vi "AC_Disconnect_Powerstage_v1.vi"() -> (0 "error out":errorcluster, 3 "output string":string)   [LabVIEW 2022 SP3]
uses:
  <vilib>/Instr/_visa.llb/VISA Flush IO Buffer Mask.ctl
  <vilib>/DAQmx/write.llb/DAQmx Write (Digital 1D Bool NChan 1Samp 1Line).vi
  <vilib>/DAQmx/miscellaneous.llb/DAQmx Fill In Error Info.vi
panel:
  in  "error in (no error)":errorcluster
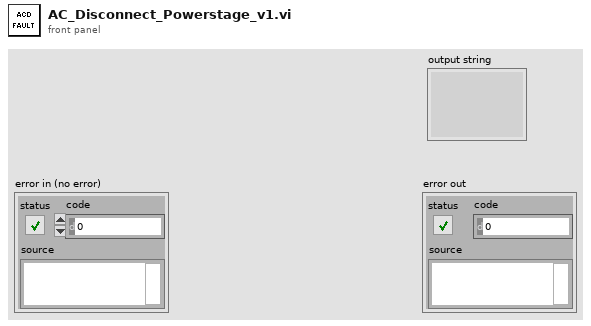
[diagram p1: front panel]
types:
  T1 = typedef "VISA Flush IO Buffer Mask.ctl" = u16
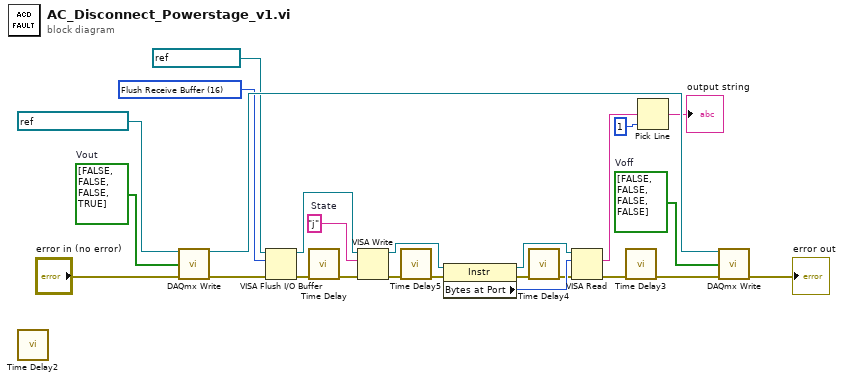
[diagram p0: block diagram]
diagram:
  w11 = "j"  # State
  w10 = bool[] [FALSE, FALSE, FALSE, FALSE]  # Voff
  w12 = bool[] [FALSE, FALSE, FALSE, TRUE]  # Vout
  w15 = T1 16 items=["Flush Receive Buffer"=16, "Write Transmit Buffer to Device"=32, "Flush Receive Buffer (No I/O)"=64, "Flush Transmit Buffer"=128] ("Mask")
  n1 = call "Time Delay2"() -> ()  [unwired: 11 in, 1 out]
  n2 = call-poly <vilib>:"DAQmx Write.vi"("task/channels in"=refnum<k21> "FTS2_DigitalOut", "data"=w12, "error in"="error in (no error)") -> ("task out"=w21:refnum<k21>, "error out"=w13:errorcluster)  [unwired: 10 in, 1 out]
  n3 = VISA Flush I/O Buffer(VISA resource name=refnum<visa-resource-name> "ControlBoard", mask (16)=w15, error in (no error)=w13) -> (VISA resource name out=w17:refnum<visa-resource-name>, error out=w14:errorcluster)
  n4 = call "Time Delay"("error in (no error)"=w14) -> ("error out"=w25:errorcluster)  [unwired: 10 in]
  n5 = VISA Write(VISA resource name=w17, write buffer=w11, error in (no error)=w25) -> (VISA resource name out=w20:refnum<visa-resource-name>, error out=w7:errorcluster)  [unwired: 1 out]
  n6 = call "Time Delay5"("error in (no error)"=w7) -> ("error out"=w6:errorcluster)  [unwired: 10 in]
  n7 = property class="Instr"(reference=w20, error in=w6) -> (reference out=w19:refnum<visa-resource-name>, error out=w5:errorcluster, "Bytes at Port"=w18:u32)
  n8 = call "Time Delay4"("error in (no error)"=w5) -> ("error out"=w4:errorcluster)  [unwired: 10 in]
  n9 = VISA Read(VISA resource name=w19, byte count=w18, error in (no error)=w4) -> (read buffer=w3:string, error out=w23:errorcluster)  [unwired: 2 out]
  n10 = call "Time Delay3"("error in (no error)"=w23) -> ("error out"=w22:errorcluster)  [unwired: 10 in]
  n11 = Pick Line(multi-line string=w3, line index=1) -> (output string=→"output string":string)  [unwired: 1 in]
  n12 = call-poly <vilib>:"DAQmx Write.vi"("task/channels in"=w21, "data"=w10, "error in"=w22) -> ("error out"=→"error out":errorcluster)  [unwired: 10 in, 2 out]
